vi "is_boolean_control.vi"(8 "error in (no error)":errorcluster, 11 "CMD Ring Value":string[](array[string])) -> (0 "error out":errorcluster, 2 "Is Boolean":bool, 3 "CMD Ring Value Out":string[](array[string]))   [LabVIEW 2018]
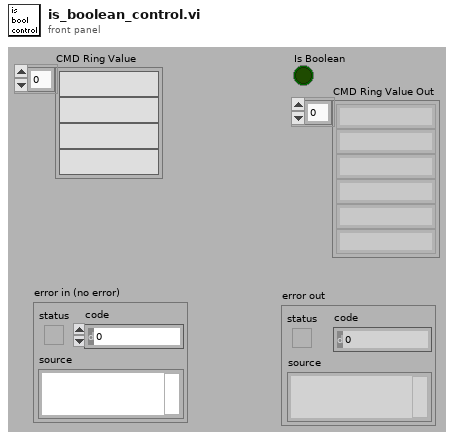
[diagram p1: front panel]
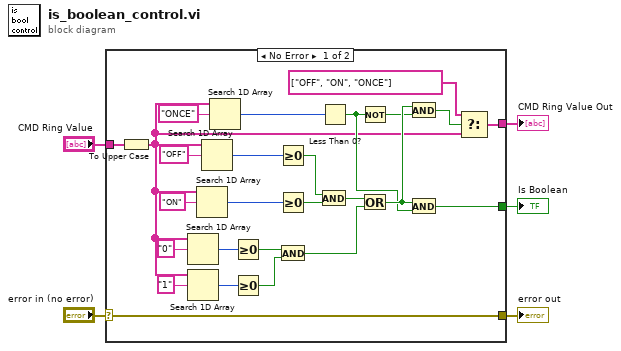
[diagram p0: block diagram]
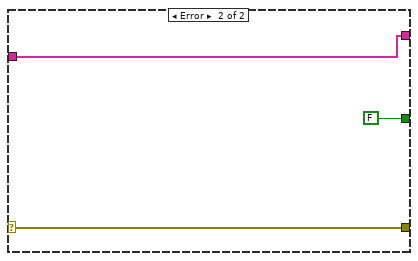
[diagram p2: hidden frame]
diagram:
  n1 = case shown="No Error" "error in (no error)" {
    selector: "error in (no error)" -> [w16 w34]
    tunnel: "CMD Ring Value" -> [w30 w32]
    tunnel: [w13 FALSE] -> w4
    tunnel: [w16 w34] -> w2
    tunnel: [w6 w32] -> w1
    frame No Error {
      n2 = To Upper Case(1:w30) -> (0:w7:string[])
      n3 = Search 1D Array(1D array=w7, element="0") -> (index of element=w24:i32)  [unwired: 1 out]
      n4 = Search 1D Array(1D array=w7, element="1") -> (index of element=w23:i32)  [unwired: 1 out]
      n5 = Search 1D Array(1D array=w7, element="ON") -> (index of element=w25:i32)  [unwired: 1 out]
      n6 = Search 1D Array(1D array=w7, element="OFF") -> (index of element=w26:i32)  [unwired: 1 out]
      n7 = Search 1D Array(1D array=w7, element="ONCE") -> (index of element=w14:i32)  [unwired: 1 out]
      n8 = Greater Or Equal To 0?(x=w24) -> (x >= 0?=w20:bool)
      n9 = Greater Or Equal To 0?(x=w23) -> (x >= 0?=w19:bool)
      n10 = Greater Or Equal To 0?(x=w26) -> (x >= 0?=w22:bool)
      n11 = Greater Or Equal To 0?(x=w25) -> (x >= 0?=w21:bool)
      n12 = And(x=w20, y=w19) -> (x .and. y?=w17:bool)
      n13 = And(x=w22, y=w21) -> (x .and. y?=w18:bool)
      n14 = Less Than 0?(x=w14) -> (x < 0?=w11:bool)
      n15 = Not(x=w11) -> (.not. x?=w10:bool)
      n16 = Or(x=w18, y=w17) -> (x .or. y?=w12:bool)
      n17 = And(x=w12, y=w10) -> (x .and. y?=w9:bool)
      n18 = And(x=w12, y=w11) -> (x .and. y?=w13:bool)
      n19 = Select(t=string[] ["OFF", "ON", "ONCE"] ("all upper case string"), s=w9, f=w7) -> (s? t:f=w6:string[])
    }
    frame Error {
    }
  }
  "Is Boolean" <- w4
  "error out" <- w2
  "CMD Ring Value Out" <- w1
